vi "_Run Engine.vi"() -> ()   [LabVIEW 2015]
uses:
  Type/_Run State.ctl
  Type/_Data Operation.ctl
  Type/_File Command.ctl
  Type/_RT Command.ctl
  Configuration/_Global Configuration.vi
  Server/_Server Global.vi
panel:
  out "size(s)":i32
  out "first subarray":i32[](array[numeric])
  out "error":string
  out "Occurance timed out":bool
  out "Done":bool
  out "error out":errorcluster
  out "Remaining Scans":i32
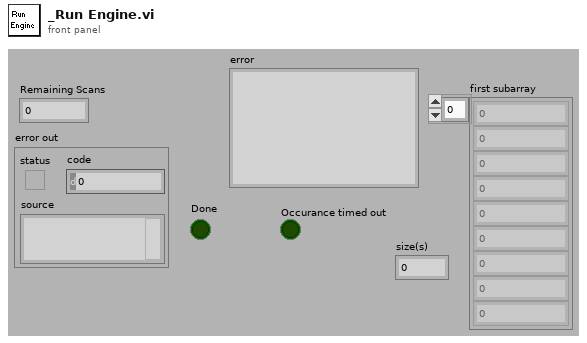
[diagram p1: front panel]
types:
  T1 = typedef "_Run State.ctl" = enum16{"Init", "Update", "Start", "End", "Error"}
  T2 = typedef "_Data Operation.ctl" = enum8{"Initialize", "Get Data", "Set Data", "Close"}
  T3 = typedef "_File Command.ctl" = enum16{"No Command", "Open", "Open Read", "Write", "Get Spectrum", "Close"}
  T4 = typedef "_RT Command.ctl" = enum16{"xml Start Run", "xml Start Actual Run", "xml Stop Run", "xml Runtime Update", "xml Get Status", "xml Get Table", "xml Set Table", "xml Get Configuration", "xml System Status", "xml Set LC Input Logic", "xml Get Data", "xml Get Info", "Start", "StartActualRun", "Stop", "Runtime Update", "Get Data", "Get Info", "Get Status", "Get Param", "Get Config", "Get Table", "Read ADC", "Set Oscillator", "Update Config", "Update Table", "Set All Pol", "Set Pol and DC", "Set Max Mass", "Toggle RP", "Toggle EL", "Set PIC", "Initialize Turbo", "Send Turbo Comm", "Close Turbo", "P1", "P2", "P3", "Send Serial", "Set LC Out", "Get LC In", "Read VAC", "Test Table", "Toggle Power", "Get Startup", "Set Startup", "Get ADC Table", "Set ADC Table", "Get Brief Status", "Get Detail Status", "Auxiliary Update", "Set CC Logics", "Set CC Input Logics", "Ignore Error", "invalid"}
  T5 = typedef "_XML Expt.ctl" = cluster{"StartT(mS)":i32, "#Cycles":i32, "PauseT(uS)":i32, "ScanType":i32, "Polarity":u8, "FixedMass":dbl, "DelayT(mS)":i32, "Active Ch":T6[], "Mass Range":T7[]}
  T6 = typedef "_XML Lens.ctl" = cluster{"Value":dbl, "ChID":u8}
  T7 = typedef "_Mass Range Property.ctl" = cluster{"Start":dbl, "Stop":dbl, "Step Size":dbl, "Steps":i32, "Dwell":dbl, "Parameters":T8[], "Res":T9}
  T8 = typedef "_Mass Range Parameters.ctl" = cluster{"Name":string, "Ch#":u8, "StartV":dbl, "StopV":dbl, "StepV":dbl, "Index":u8}
  T9 = typedef "_RT Res Type.ctl" = u16
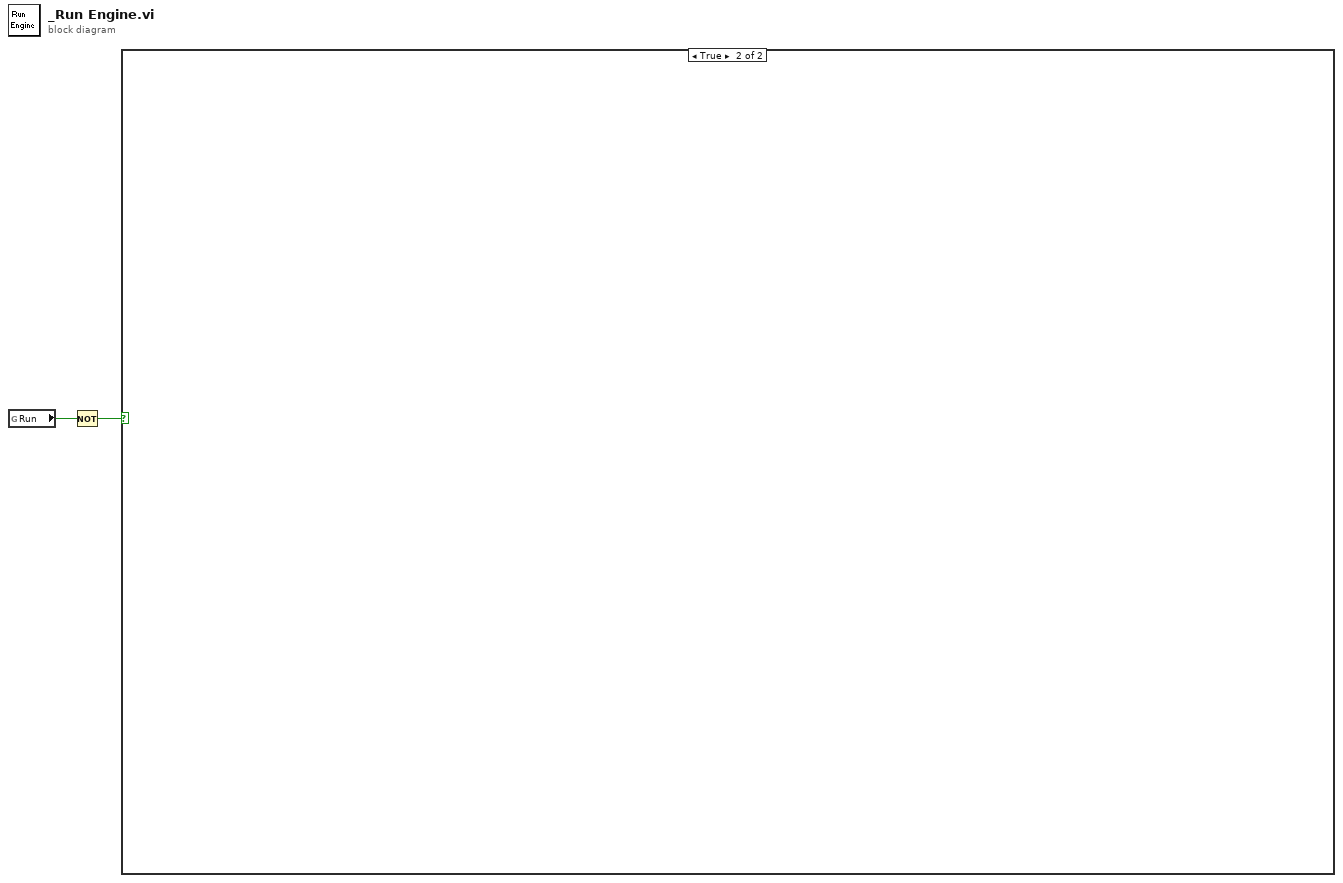
[diagram p0: block diagram]
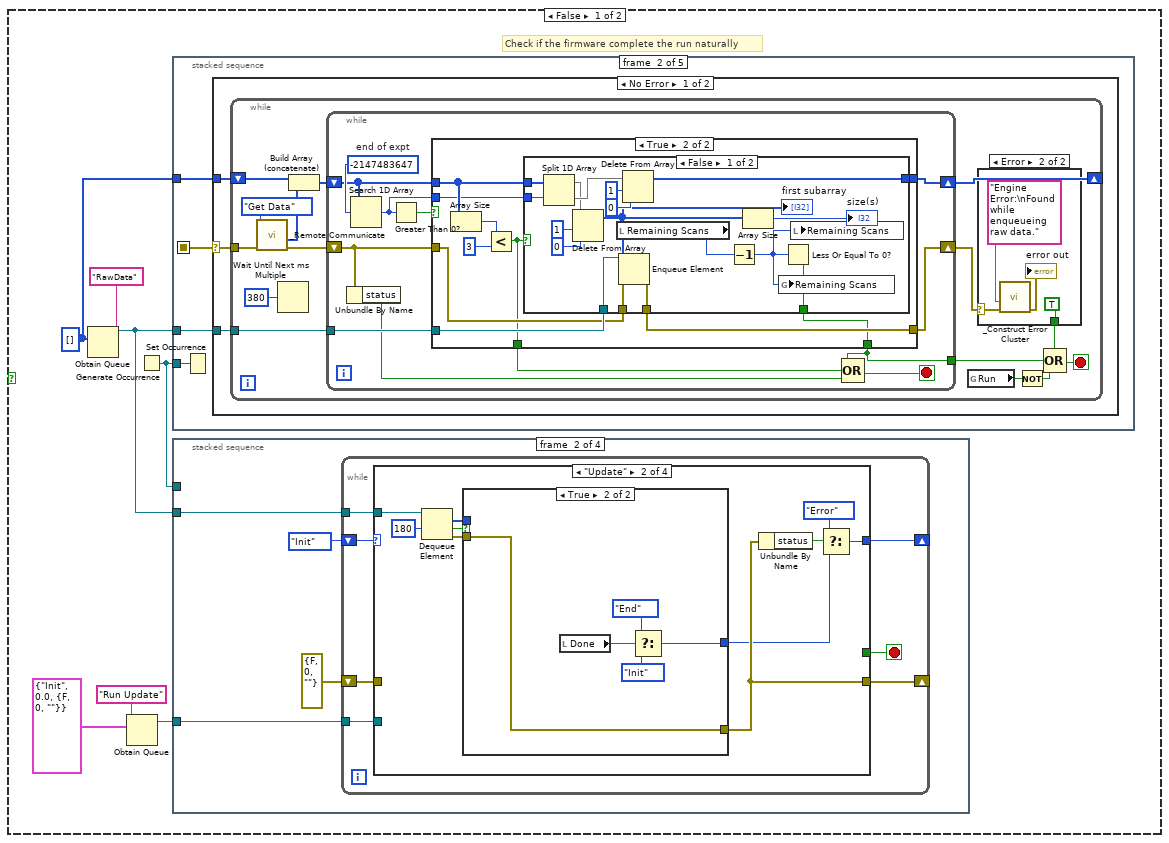
[diagram p2: hidden frame]
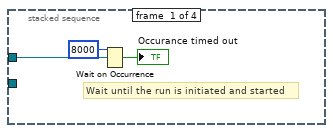
[diagram p3: hidden frame]
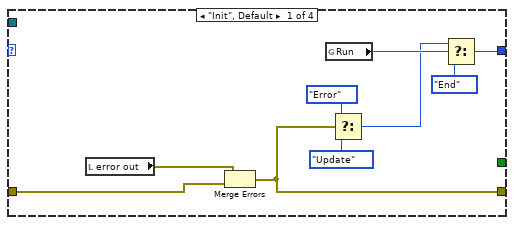
[diagram p4: hidden frame]
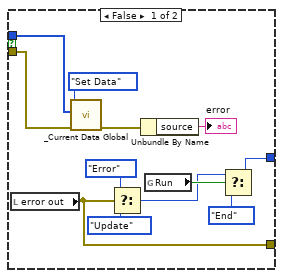
[diagram p5: hidden frame]
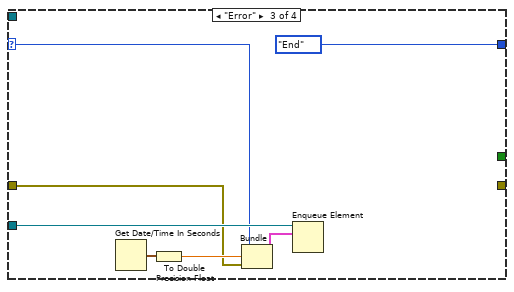
[diagram p6: hidden frame]
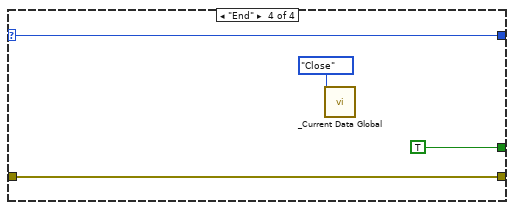
[diagram p7: hidden frame]
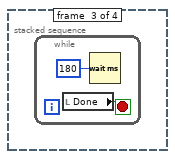
[diagram p8: hidden frame]
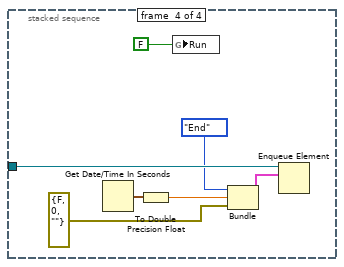
[diagram p9: hidden frame]
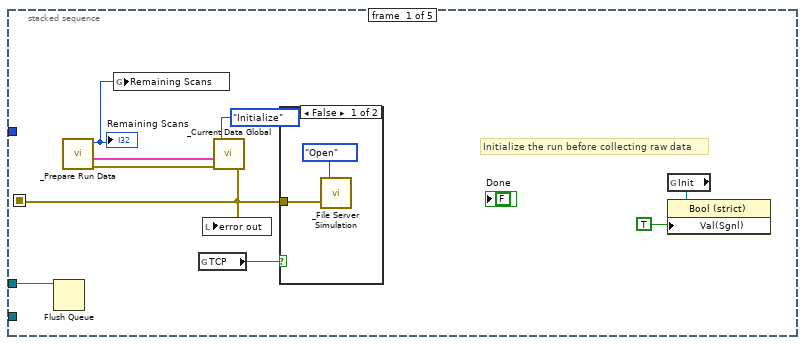
[diagram p10: hidden frame]
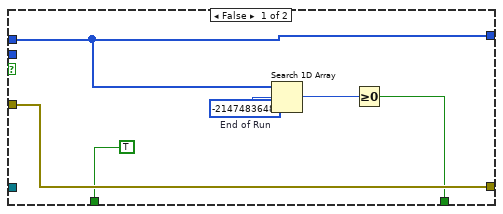
[diagram p12: hidden frame]
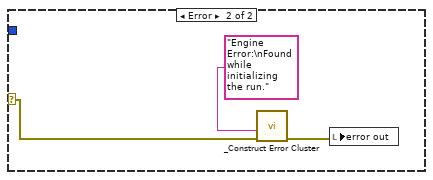
[diagram p15: hidden frame]
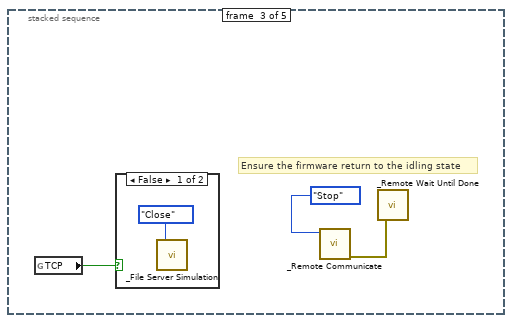
[diagram p16: hidden frame]
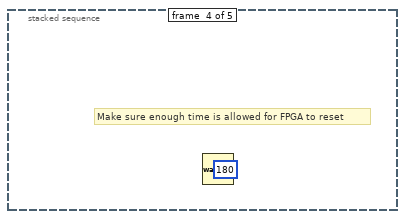
[diagram p18: hidden frame]
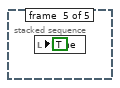
[diagram p19: hidden frame]
diagram:
  n1 = global read "_Global Configuration.vi" "Run"() -> (w2:bool)
  n2 = Not(x=w2) -> (.not. x?=w1:bool)
  n3 = case shown="True" w1 {
    frame False {
      w6 = i32[] []
      # "Check if the firmware complete the run naturally"
      n4 = Obtain Queue(name (unnamed)="RawData", element data type=w6) -> (queue out=w7:refnum<queue>)  [unwired: 3 in, 2 out]
      n5 = Obtain Queue(name (unnamed)="Run Update", element data type=cluster{T1, dbl, "error out":errorcluster} {enum."Init", 0.0, "error out"={"status"=FALSE, "code"=0, "source"=""}}) -> (queue out=w4:refnum<queue>)  [unwired: 3 in, 2 out]
      n6 = Generate Occurrence() -> (w8:refnum<k4>)
      n7 = stacked-sequence {
        seq-local: [w80 _ _ _ _] -> [_ w93 _ _ _]
        tunnel: w8 -> [_ w94 _ _ _]
        tunnel: w7 -> [w89 w95 _ _ _]
        tunnel: w6 -> [_ w92 _ _ _]
        frame #0 {
          # "Initialize the run before collecting raw data"
          n8 = Flush Queue(queue=w89) -> ()  [unwired: 1 in, 3 out]
          n9 = call "_Prepare Run Data.vi"() -> ("error out"=w84:errorcluster, "AcqMethod"=w83:T5[], "Scans"=w82:i32)  [unwired: 1 in, 8 out]
          "Remaining Scans" <- w82
          n10 = global write "_Server Global.vi" "Remaining Scans"(w82) -> ()
          n11 = global read "_Global Configuration.vi" "TCP"() -> (w81:bool)
          n12 = call "_Current Data Global.vi"("error in (no error)"=w84, "AcqMethod"=w83, "Operation"=_Data_Operation."Initialize") -> ("error out"=w80:errorcluster)  [unwired: 1 in, 3 out]
          n13 = local write "error out"(w80) -> ()
          n14 = case shown="False" w81 {
            tunnel: w80 -> [w90 _]
            frame False {
              n15 = call "_File Server Simulation.vi"("ErrorIn"=w90, "FileCommand"=_File_Command."Open") -> ()  [unwired: 2 out]
            }
            frame True {
            }
          }
          n16 = global read "_Global Configuration.vi" "Init"() -> (w87:refnum<vi>)
          n17 = property class="Bool (strict)"(reference=w87, "Val(Sgnl)"=TRUE ("Value (Signaling)")) -> ()  [unwired: 1 in, 2 out]
          "Done" <- FALSE ("Done")
        }
        frame #1 {
          n18 = Set Occurrence(w94) -> ()
          n19 = case shown="No Error" w93 {
            selector: w93 -> [w97 w165]
            tunnel: w95 -> [w98 _]
            tunnel: w92 -> [w96 _]
            frame No Error {
              n20 = while {
                tunnel: w98 -> [w112]
                tunnel: w97 -> [w108]
                shift-right: [w105] -> _
                shift-left: w96 -> [w103]
                stop <- w111 stop-if-true
                n21 = call "_Remote Communicate.vi"("error in (no error)"=w108, "Command"=_RT_Command."Get Data") -> ("error out"=w101:errorcluster, "Data Array"=w100:i32[])  [unwired: 4 in, 2 out]
                n22 = Wait Until Next ms Multiple(millisecond multiple=u32 380) -> ()  [unwired: 1 out]
                n23 = Build Array (concatenate)(w103, w100) -> (w102:i32[])
                n24 = while {
                  tunnel: w112 -> [w125]
                  tunnel: [w117] -> w104
                  shift-right: [w123] -> w105
                  shift-left: w102 -> [w121]
                  shift-right: [w124] -> w107
                  shift-left: w101 -> [w119]
                  stop <- w115 stop-if-true
                  w122 = -2147483647  # end of expt
                  n25 = Unbundle By Name(w119) -> ("status"=w116:bool)
                  n26 = Search 1D Array(1D array=w121, element=w122) -> (index of element=w120:i32)  [unwired: 1 out]
                  n27 = Greater Than 0?(x=w120) -> (x > 0?=w118:bool)
                  n28 = case shown="True" w118 {
                    tunnel: w119 -> [w131 w139]
                    tunnel: w125 -> [_ w140]
                    tunnel: [w131 w138] -> w124
                    tunnel: w121 -> [w128 w134]
                    tunnel: [w128 w141] -> w123
                    tunnel: [w127 w137] -> w117
                    tunnel: w120 -> [_ w133]
                    tunnel: [TRUE w132] -> w114
                    frame False {
                      w129 = -2147483648  # End of Run
                      n29 = Search 1D Array(1D array=w128, element=w129) -> (index of element=w130:i32)  [unwired: 1 out]
                      n30 = Greater Or Equal To 0?(x=w130) -> (x >= 0?=w127:bool)
                    }
                    frame True {
                      n31 = Array Size(array=w134) -> (size(s)=w136:i32)
                      n32 = Less?(x=w136, y=3) -> (x < y?=w132:bool)
                      n33 = case shown="False" w132 {
                        tunnel: w134 -> [w158 w159]
                        tunnel: w133 -> [w157 _]
                        tunnel: [w151 w159] -> w141
                        tunnel: w140 -> [w142 _]
                        tunnel: w139 -> [w153 w160]
                        tunnel: [w152 w160] -> w138
                        tunnel: [w144 _] -> w137
                        frame False {
                          n34 = Split 1D Array(array=w158, index=w157) -> (first subarray=w146:i32[], second subarray=w155:i32[])
                          n35 = Delete From Array(array=w146, length=1, index=0) -> (array with subset deleted=w145:i32[])  [unwired: 1 out]
                          "first subarray" <- w145
                          n36 = local read "Remaining Scans"() -> (w150:i32)
                          n37 = Enqueue Element(queue=w142, element=w145, error in (no error)=w153) -> (error out=w152:errorcluster)  [unwired: 3 out]
                          n38 = Delete From Array(array=w155, length=1, index=0) -> (array with subset deleted=w151:i32[])  [unwired: 1 out]
                          n39 = Decrement(x=w150) -> (x-1=w143:i32)
                          n40 = Array Size(array=w145) -> (size(s)=→"size(s)":i32)
                          n41 = global write "_Server Global.vi" "Remaining Scans"(w143) -> ()
                          n42 = Less Or Equal To 0?(x=w143) -> (x <= 0?=w144:bool)
                          n43 = local write "Remaining Scans"(w143) -> ()
                        }
                        frame True {
                        }
                      }
                    }
                  }
                  n44 = Compound Arithmetic op=OR(w117, w114, w116) -> (w115:bool)
                }
                n45 = global read "_Global Configuration.vi" "Run"() -> (w110:bool)
                n46 = case shown="Error" w107 {
                  selector: w107 -> [_ w164]
                  tunnel: [_ TRUE] -> w106
                  frame No Error {
                  }
                  frame Error {
                    n47 = call "_Construct Error Cluster.vi"("error in"=w164, "reason"="Engine Error:\nFound while enqueueing raw data." ("format string")) -> ("error out"=→"error out":errorcluster)  [unwired: 2 in, 3 out]
                  }
                }
                n48 = Not(x=w110) -> (.not. x?=w109:bool)
                n49 = Compound Arithmetic op=OR(w106, w104, w109) -> (w111:bool)
              }
            }
            frame Error {
              n50 = call "_Construct Error Cluster.vi"("error in"=w165, "reason"="Engine Error:\nFound while initializing the run." ("format string")) -> ("error out"=w166:errorcluster)  [unwired: 2 in, 3 out]
              n51 = local write "error out"(w166) -> ()
            }
          }
        }
        frame #2 {
          # "Ensure the firmware return to the idling state"
          n52 = global read "_Global Configuration.vi" "TCP"() -> (w168:bool)
          n53 = case shown="False" w168 {
            frame False {
              n54 = call "_File Server Simulation.vi"("FileCommand"=_File_Command."Close") -> ()  [unwired: 1 in, 2 out]
            }
            frame True {
            }
          }
          n55 = call "_Remote Communicate.vi"("Command"=_RT_Command."Stop") -> ("error out"=w170:errorcluster)  [unwired: 5 in, 3 out]
          n56 = call "_Remote Wait Until Done.vi"("error IO"=w170) -> ()  [unwired: 1 in, 2 out]
        }
        frame #3 {
          # "Make sure enough time is allowed for FPGA to reset"
          n57 = Wait (ms)(milliseconds to wait=u32 180) -> ()  [unwired: 1 out]
        }
        frame #4 {
          n58 = local write "Done"(TRUE ("Done")) -> ()
        }
      }
      n59 = stacked-sequence {
        tunnel: w8 -> [w12 _ _ _]
        tunnel: w7 -> [_ w15 _ _]
        tunnel: w4 -> [_ w14 _ w76]
        frame #0 {
          # "Wait until the run is initiated and started"
          n60 = Wait on Occurrence(2:w12, 3:8000 ("ms timeout (-1)")) -> (0:→"Occurance timed out":bool)  [unwired: 1 out]
        }
        frame #1 {
          n61 = while {
            shift-right: [w22] -> _
            shift-left: _Run_State."Init" -> [w23]
            shift-right: [w21] -> _
            shift-left: errorcluster {"status"=FALSE, "code"=0, "source"=""} ("error out") -> [w20]
            tunnel: w14 -> [w18]
            tunnel: w15 -> [w17]
            stop <- w19 stop-if-true
            n62 = case shown="\"Update\"" w23 {
              selector: w23 -> [_ _ w61 w69]
              tunnel: [w26 w40 _Run_State."End" w69] -> w22
              tunnel: [w29 w34 _ w68] -> w21
              tunnel: w20 -> [w31 _ w60 w68]
              tunnel: [_ _ _ TRUE] -> w19
              tunnel: w18 -> [_ _ w62 _]
              tunnel: w17 -> [_ w39 _ _]
              frame "Init", Default {
                n63 = local read "error out"() -> (w30:errorcluster)
                n64 = Merge Errors(w30, w31) -> (w29:errorcluster)
                n65 = global read "_Global Configuration.vi" "Run"() -> (w25:bool)
                n66 = Select(t=_Run_State."Error", s=w29, f=_Run_State."Update") -> (s? t:f=w24:T1)
                n67 = Select(t=w24, s=w25, f=_Run_State."End") -> (s? t:f=w26:T1)
              }
              frame "Update" {
                n68 = Dequeue Element(queue=w39, timeout in ms (-1)=180) -> (element=w35:i32[], timed out?=w37:bool, error out=w36:errorcluster)  [unwired: 1 in, 1 out]
                n69 = case shown="True" w37 {
                  tunnel: w36 -> [w46 w59]
                  tunnel: w35 -> [w45 _]
                  tunnel: [w47 w59] -> w34
                  tunnel: [w48 w55] -> w33
                  frame False {
                    n70 = local read "error out"() -> (w47:errorcluster)
                    n71 = call "_Current Data Global.vi"("error in (no error)"=w46, "Spectrum in"=w45, "Operation"=_Data_Operation."Set Data") -> ("error out"=w43:errorcluster)  [unwired: 1 in, 3 out]
                    n72 = Select(t=_Run_State."Error", s=w47, f=_Run_State."Update") -> (s? t:f=w49:T1)
                    n73 = Unbundle By Name(w43) -> ("source"=→"error":string)
                    n74 = global read "_Global Configuration.vi" "Run"() -> (w50:bool)
                    n75 = Select(t=w49, s=w50, f=_Run_State."End") -> (s? t:f=w48:T1)
                  }
                  frame True {
                    n76 = local read "Done"() -> (w58:bool)
                    n77 = Select(t=_Run_State."End", s=w58, f=_Run_State."Init") -> (s? t:f=w55:T1)
                  }
                }
                n78 = Unbundle By Name(w34) -> ("status"=w41:bool)
                n79 = Select(t=_Run_State."Error", s=w41, f=w33) -> (s? t:f=w40:T1)
              }
              frame "Error" {
                n80 = Get Date/Time In Seconds() -> (seconds since 1Jan1904=w65:timestamp)
                n81 = To Double Precision Float(number=w65) -> (double precision float=w63:dbl)
                n82 = Bundle(w61, w63, "error out"=w60) -> (w64:cluster{T1, dbl, "error out":errorcluster})  [unwired: 1 out]
                n83 = Enqueue Element(queue=w62, element=w64) -> ()  [unwired: 1 in, 4 out]
              }
              frame "End" {
                n84 = call "_Current Data Global.vi"("Operation"=_Data_Operation."Close") -> ()  [unwired: 3 in, 4 out]
              }
            }
          }
        }
        frame #2 {
          n85 = while {
            stop <- w72 stop-if-true
            n86 = local read "Done"() -> (w72:bool)
            n87 = Wait (ms)(milliseconds to wait=u32 180) -> ()  [unwired: 1 out]
          }
        }
        frame #3 {
          n88 = Get Date/Time In Seconds() -> (seconds since 1Jan1904=w79:timestamp)
          n89 = To Double Precision Float(number=w79) -> (double precision float=w77:dbl)
          n90 = global write "_Global Configuration.vi" "Run"(FALSE ("Update")) -> ()
          n91 = Bundle(_Run_State."End", w77, "error out"=errorcluster {"status"=FALSE, "code"=0, "source"=""}) -> (w78:cluster{T1, dbl, "error out":errorcluster})  [unwired: 1 out]
          n92 = Enqueue Element(queue=w76, element=w78) -> ()  [unwired: 1 in, 4 out]
        }
      }
    }
    frame True {
    }
  }
